vi "Set_Parameter_Instrument (Json).vi"(8 "error in (no error)":errorcluster caption="entrée d'erreur (pas d'erreur)", 10 "Parameter (Json)":string, 11 "Show_Information en entrée":refnum<class "Operator_Information.lvclass">) -> (0 "error out":errorcluster caption="sortie d'erreur", 3 "Show_Information en sortie":refnum<class "Operator_Information.lvclass">)   [LabVIEW 2020, in "Library Test.lvlib" / "Operator_Information.lvclass"]
uses:
  Operator_Information.lvclass
  C:/Users/ngarcin/OneDrive - Altyor/Standard TB/Class/Test/Test (Default)/Test (Default).lvclass
  Operator_Information.lvclass/Operator_Information.ctl
  JSON API/JSON Value/Set from JSON string.vi
  Test_Without_Instr/Test_Without_Inst.lvclass
  JSON API/JSON Value/JSON Value.lvclass
  JSON API/Variant JSON/Variant JSON.lvlib
  JSON API/Get Polymorphic/JSON GetSet.lvlib
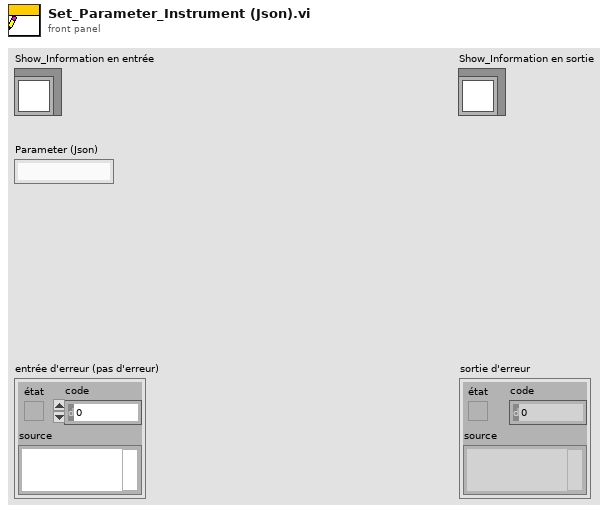
[diagram p1: front panel]
types:
  T1 = cluster{"Information_Operator":string, "Path_Picture":path}
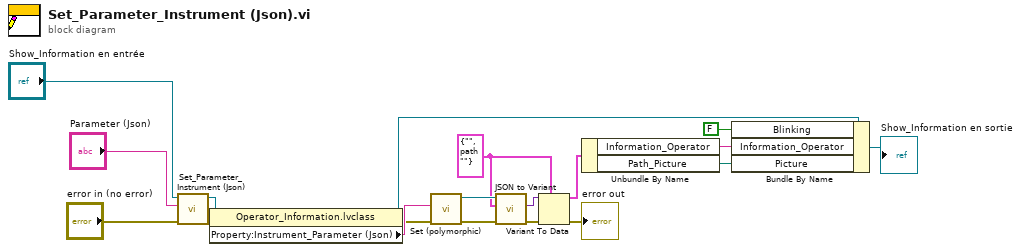
[diagram p0: block diagram]
diagram:
  w4 = T1 {"Information_Operator"="", "Path_Picture"=path ""} ("Cluster des données privées de classe")
  n1 = call-parent "Set_Parameter_Instrument (Json).vi"("error in (no error)"="error in (no error)", "Parameter (Json)"="Parameter (Json)", "Test (Default) en entrée"="Show_Information en entrée") -> ("error out"=w9:errorcluster, "Test (Default) en sortie"=w10:refnum<class "Operator_Information.lvclass">)  [unwired: 7 in]
  n2 = property class="Operator_Information.lvclass"(reference=w10, error in=w9) -> (reference out=w8:refnum<class "Operator_Information.lvclass">, error out=w15:errorcluster, "Property:Instrument_Parameter (Json)"=w16:string)
  n3 = call-poly "Set (polymorphic).vi"("error in (no error)"=w15, "JSON stream"=w16) -> ("error out"=w12:errorcluster, "JSON Value out"=w14:refnum<class "JSON Value.lvclass">)  [unwired: 7 in, 1 out]
  n4 = call "JSON to Variant.vi"("error in (no error)"=w12, "Variant (Data Type)"=w4, "JSON Value"=w14) -> ("error out"=w13:errorcluster, "Variant out"=w11:variant)  [unwired: 7 in]
  n5 = Variant To Data(error in=w13, type=w4, Variant=w11) -> (data=w7:T1, error out=→"error out":errorcluster)
  n6 = Unbundle By Name(w7) -> ("Information_Operator"=w6:string, "Path_Picture"=w5:path)
  n7 = Bundle By Name(cluster=w8, "Blinking"=FALSE ("Ok_Button_Visible"), "Information_Operator"=w6, "Picture"=w5) -> (→"Show_Information en sortie":refnum<class "Operator_Information.lvclass">)
